vi "Tester.vi"() -> ()   [LabVIEW 2017]
uses:
  myEmptyClass/myEmptyClass.lvclass
  myOtherClass/myOtherClass.lvclass
  myChildClass/myChildClass.lvclass
  Z:/Code/Git/WC/Insert LVClass Property Node/tests/myClass/myClass.lvclass
  myChildClass/myChildClass.lvclass/myChildClass.ctl
  myClass/myClass.lvclass/myClass.ctl
  myOtherClass/myOtherClass.lvclass/myOtherClass.ctl
  myChildClass/Write Boolean.vi
  myChildClass/Write Numeric.vi
  myChildClass/Write String.vi
  myClass/Write Class Entry.vi
  myChildClass/Read Boolean.vi
  myChildClass/Read Numeric.vi
  myChildClass/Read String.vi
  myClass/Read Class Entry.vi
  myOtherClass/Write Read and Write.vi
  myOtherClass/Write Write.vi
  myOtherClass/Read Read.vi
  myOtherClass/Read Read and Write.vi
panel:
  out "Numeric 2":dbl
  out "String 2":string
  out "Class Entry 2":refnum<class "myEmptyClass.lvclass">
  out "Boolean 2":bool
  out "Read and Write 2":bool
  out "Read 2":bool
  out "Class Entry":refnum<class "myEmptyClass.lvclass">
  out "String":string
  out "Numeric":dbl
  out "Boolean":bool
  out "Read":bool
  out "Read and Write":bool
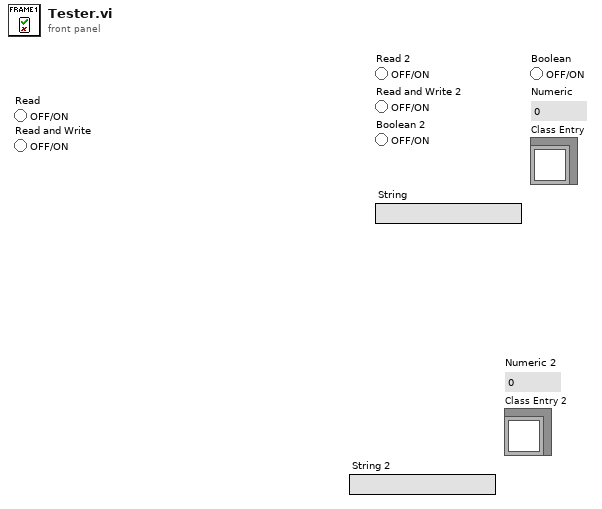
[diagram p1: front panel]
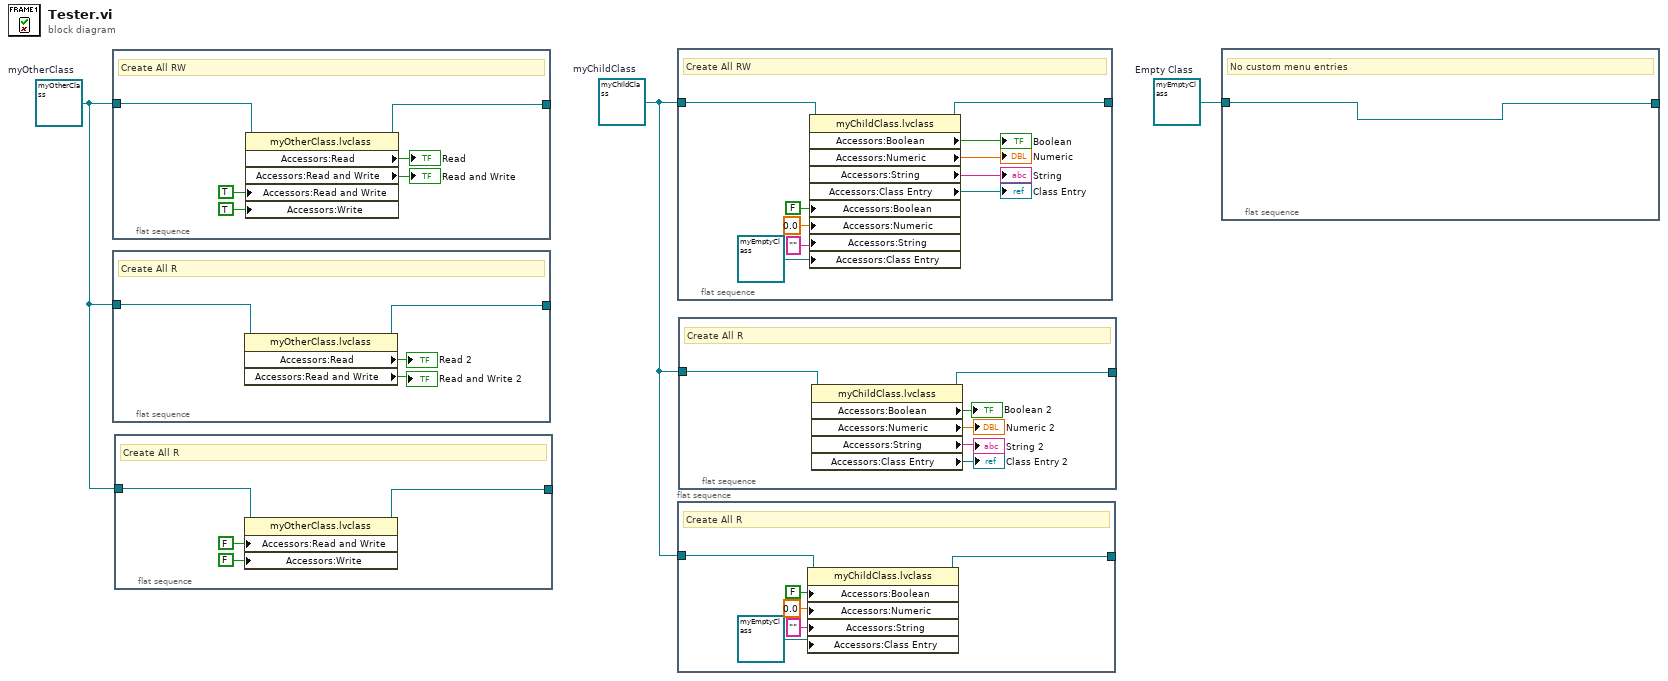
[diagram p0: block diagram]
diagram:
  w1 = refnum<class "myEmptyClass.lvclass"> refnum  # Empty Class
  w2 = refnum<class "myChildClass.lvclass"> refnum  # myChildClass
  w3 = refnum<class "myOtherClass.lvclass"> refnum  # myOtherClass
  n1 = flat-sequence {
    tunnel: w3 -> [w4]
    tunnel: [w9] -> _
    frame #0 {
      # "Create All RW"
      n2 = property class="myOtherClass.lvclass"(reference=w4, "Accessors:Read and Write"=TRUE ("Read and Write"), "Accessors:Write"=TRUE ("Write")) -> (reference out=w9:refnum<class "myOtherClass.lvclass">, "Accessors:Read"=→"Read":bool, "Accessors:Read and Write"=→"Read and Write":bool)  [unwired: 1 in, 1 out]
    }
  }
  n3 = flat-sequence {
    tunnel: w3 -> [w13]
    tunnel: [w12] -> _
    frame #0 {
      # "Create All R"
      n4 = property class="myOtherClass.lvclass"(reference=w13) -> (reference out=w12:refnum<class "myOtherClass.lvclass">, "Accessors:Read"=→"Read 2":bool, "Accessors:Read and Write"=→"Read and Write 2":bool)  [unwired: 1 in, 1 out]
    }
  }
  n5 = flat-sequence {
    tunnel: w3 -> [w17]
    tunnel: [w16] -> _
    frame #0 {
      # "Create All R"
      n6 = property class="myOtherClass.lvclass"(reference=w17, "Accessors:Read and Write"=FALSE ("Read and Write"), "Accessors:Write"=FALSE ("Write")) -> (reference out=w16:refnum<class "myOtherClass.lvclass">)  [unwired: 1 in, 1 out]
    }
  }
  n7 = flat-sequence {
    tunnel: w2 -> [w27]
    tunnel: [w26] -> _
    frame #0 {
      # "Create All RW"
      n8 = property class="myChildClass.lvclass"(reference=w27, "Accessors:Boolean"=FALSE ("Boolean"), "Accessors:Numeric"=0.0 ("Numeric"), "Accessors:String"="" ("String"), "Accessors:Class Entry"=refnum<class "myEmptyClass.lvclass"> refnum ("Class Entry")) -> (reference out=w26:refnum<class "myChildClass.lvclass">, "Accessors:Boolean"=→"Boolean":bool, "Accessors:Numeric"=→"Numeric":dbl, "Accessors:String"=→"String":string, "Accessors:Class Entry"=→"Class Entry":refnum<class "myEmptyClass.lvclass">)  [unwired: 1 in, 1 out]
    }
  }
  n9 = flat-sequence {
    tunnel: w2 -> [w33]
    tunnel: [w32] -> _
    frame #0 {
      # "Create All R"
      n10 = property class="myChildClass.lvclass"(reference=w33, "Accessors:Boolean"=FALSE ("Boolean"), "Accessors:Numeric"=0.0 ("Numeric"), "Accessors:String"="" ("String"), "Accessors:Class Entry"=refnum<class "myEmptyClass.lvclass"> refnum ("Class Entry")) -> (reference out=w32:refnum<class "myChildClass.lvclass">)  [unwired: 1 in, 1 out]
    }
  }
  n11 = flat-sequence {
    tunnel: w2 -> [w39]
    tunnel: [w38] -> _
    frame #0 {
      # "Create All R"
      n12 = property class="myChildClass.lvclass"(reference=w39) -> (reference out=w38:refnum<class "myChildClass.lvclass">, "Accessors:Boolean"=→"Boolean 2":bool, "Accessors:Numeric"=→"Numeric 2":dbl, "Accessors:String"=→"String 2":string, "Accessors:Class Entry"=→"Class Entry 2":refnum<class "myEmptyClass.lvclass">)  [unwired: 1 in, 1 out]
    }
  }
  n13 = flat-sequence {
    tunnel: w1 -> [w40]
    tunnel: [w40] -> _
    frame #0 {
      # "No custom menu entries"
    }
  }
